vi "Dialog Launcher.vi"(8 "error in (no error)":errorcluster, 10 "Message":string, 11 "Title":string) -> (0 "error out":errorcluster)   [LabVIEW 2023]
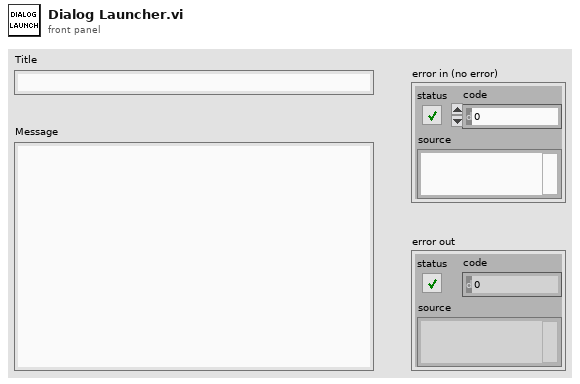
[diagram p1: front panel]
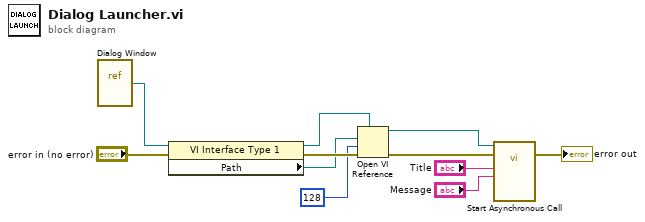
[diagram p0: block diagram]
diagram:
  n1 = vi-ref "Dialog Window.vi"() -> (w11:refnum<vi>)
  n2 = property class="VI Interface Type 1"(reference=w11, error in="error in (no error)") -> (reference out=w9:refnum<vi>, error out=w10:errorcluster, "Path"=w8:path)
  n3 = Open VI Reference(type specifier VI Refnum (for type only)=w9, vi path=w8, options=128, error in (no error)=w10) -> (vi reference=w6:refnum<vi>, error out=w7:errorcluster)  [unwired: 2 in]
  n4 = call-by-ref "Start Asynchronous Call"(reference=w6, error in=w7, "Message"="Message", "Title"="Title") -> (error out=→"error out":errorcluster)  [unwired: 10 in, 1 out]
